vi "Gas Set Setpoint_including_correction_factor.vi"(6 "Gas Set (0)":i32, 7 "Set? (F:Read)":bool, 8 "Error In":errorcluster, 9 "Setpoint (0%)":dbl, 10 "Channel (0)":i32, 11 "VISA resource name":refnum<visa-resource-name>) -> (0 "Error Out":errorcluster, 1 "Setpoint out":dbl, 3 "dup VISA resource name":refnum<visa-resource-name>)   [LabVIEW 2011, in "MGC647C.lvlib"]
doc: "Read/Set setpoint in a gas set."
uses:
  <instrlib>/MGC647C/MGC647C.lvlib
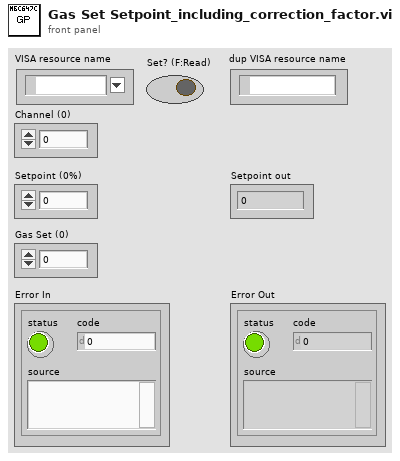
[diagram p1: front panel]
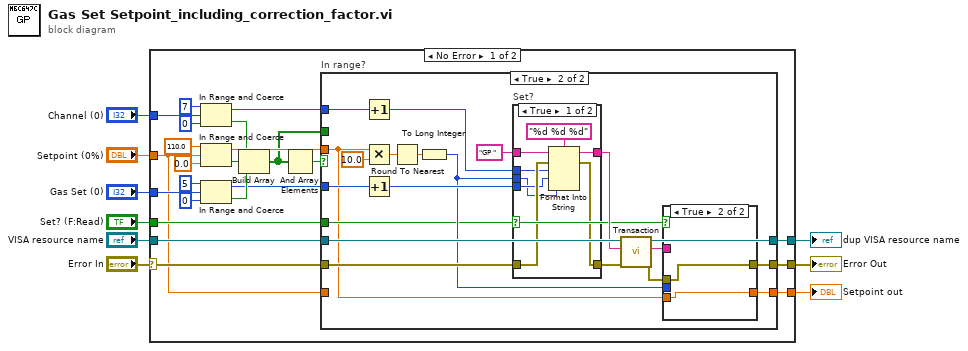
[diagram p0: block diagram]
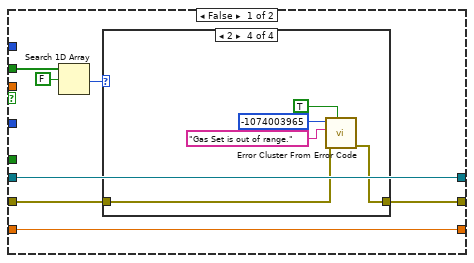
[diagram p2: hidden frame]
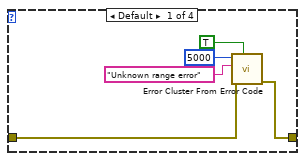
[diagram p3: hidden frame]
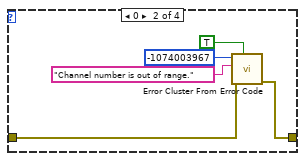
[diagram p4: hidden frame]
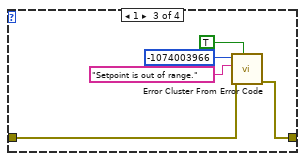
[diagram p5: hidden frame]
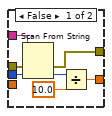
[diagram p6: hidden frame]
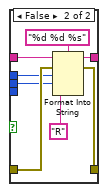
[diagram p7: hidden frame]
diagram:
  n1 = case shown="No Error" "Error In" {
    selector: "Error In" -> [w27 w106]
    tunnel: "VISA resource name" -> [w32 w105]
    tunnel: [w31 w105] -> w8
    tunnel: [w30 w106] -> w7
    tunnel: "Set? (F:Read)" -> [w29 _]
    tunnel: "Setpoint (0%)" -> [w13 w107]
    tunnel: [w26 w107] -> w1
    tunnel: "Channel (0)" -> [w23 _]
    tunnel: "Gas Set (0)" -> [w16 _]
    frame No Error {
      n2 = In Range and Coerce(upper limit=7, x=w23, lower limit=0) -> (coerced(x)=w22:i32, In Range?=w21:bool)
      n3 = In Range and Coerce(upper limit=110.0, x=w13, lower limit=0.0) -> (coerced(x)=w28:dbl, In Range?=w10:bool)
      n4 = In Range and Coerce(upper limit=5, x=w16, lower limit=0) -> (coerced(x)=w14:i32, In Range?=w15:bool)
      n5 = Build Array(w21, w10, w15) -> (w11:bool[])
      n6 = And Array Elements(Boolean array=w11) -> (logical AND=w12:bool)
      n7 = case "In range?" shown="True" w12 {
        tunnel: w32 -> [w37 w79]
        tunnel: [w37 w78] -> w31
        tunnel: [w38 w73] -> w30
        tunnel: w29 -> [_ w61]
        tunnel: w28 -> [_ w60]
        tunnel: w27 -> [w39 w77]
        tunnel: [w36 w66] -> w26
        tunnel: w22 -> [_ w72]
        tunnel: w14 -> [_ w68]
        tunnel: w13 -> [w36 _]
        tunnel: w11 -> [w35 _]
        frame False {
          n8 = Search 1D Array(1D array=w35, element=FALSE) -> (index of element=w33:i32)  [unwired: 1 in]
          n9 = case shown="2" w33 {
            tunnel: w39 -> [w44 w49 w54 w59]
            tunnel: [w43 w48 w53 w58] -> w38
            frame Default {
              n10 = call <vilib>:"Error Cluster From Error Code.vi"("show call chain? (False)"=TRUE, "error in (no error)"=w44, "error message (\"\")"="Unknown range error" ("error message (\"\")"), "error code (0)"=5000) -> ("error out"=w43:errorcluster)  [unwired: 5 in]
            }
            frame 0 {
              n11 = call <vilib>:"Error Cluster From Error Code.vi"("show call chain? (False)"=TRUE, "error in (no error)"=w49, "error message (\"\")"="Channel number is out of range." ("error message (\"\")"), "error code (0)"=-1074003967) -> ("error out"=w48:errorcluster)  [unwired: 5 in]
            }
            frame 1 {
              n12 = call <vilib>:"Error Cluster From Error Code.vi"("show call chain? (False)"=TRUE, "error in (no error)"=w54, "error message (\"\")"="Setpoint is out of range." ("error message (\"\")"), "error code (0)"=-1074003966) -> ("error out"=w53:errorcluster)  [unwired: 5 in]
            }
            frame 2 {
              n13 = call <vilib>:"Error Cluster From Error Code.vi"("show call chain? (False)"=TRUE, "error in (no error)"=w59, "error message (\"\")"="Gas Set is out of range." ("error message (\"\")"), "error code (0)"=-1074003965) -> ("error out"=w58:errorcluster)  [unwired: 5 in]
            }
          }
        }
        frame True {
          n14 = Increment(x=w72) -> (x+1=w71:i32)
          n15 = Multiply(x=w60, y=10.0) -> (x*y=w65:dbl)
          n16 = Increment(x=w68) -> (x+1=w67:i32)
          n17 = Round To Nearest(number=w65) -> (nearest integer value=w63:dbl)
          n18 = To Long Integer(number=w63) -> (32bit integer=w62:i32)
          n19 = case "Set?" shown="True" w61 {
            tunnel: w77 -> [w96 w104]
            tunnel: [w95 w103] -> w76
            tunnel: w71 -> [w94 w102]
            tunnel: w62 -> [w89 _]
            tunnel: "GP " ("string (\"\")") -> [w93 w101]
            tunnel: [w92 w100] -> w69
            tunnel: w67 -> [w90 w97]
            frame True {
              n20 = Format Into String(format string="%d %d %d", initial string=w93, error in=w96, w94, w90, w89) -> (resulting string=w92:string, error out=w95:errorcluster)
            }
            frame False {
              n21 = Format Into String(format string="%d %d %s", initial string=w101, error in=w104, w102, w97, "R") -> (resulting string=w100:string, error out=w103:errorcluster)
            }
          }
          n22 = call <instrlib>:"Transaction.vi"("Error In"=w76, "Command"=w69, "VISA resource name"=w79) -> ("Error Out"=w74:errorcluster, "Response"=w75:string, "dup VISA resource name"=w78:refnum<visa-resource-name>)  [unwired: 6 in]
          n23 = case shown="True" w61 {
            tunnel: w75 -> [w86 _]
            tunnel: w74 -> [w85 w87]
            tunnel: [w84 w87] -> w73
            tunnel: [w82 w88] -> w66
            tunnel: w62 -> [w80 _]
            tunnel: w60 -> [_ w88]
            frame False {
              n24 = Scan From String(input string=w86, error in=w85, default 1=w80) -> (error out=w84:errorcluster, output 1=w83:i32)  [unwired: 2 in, 2 out]
              n25 = Divide(x=w83, y=10.0) -> (x/y=w82:dbl)
            }
            frame True {
            }
          }
        }
      }
    }
    frame Error {
    }
  }
  "dup VISA resource name" <- w8
  "Error Out" <- w7
  "Setpoint out" <- w1
